vi "GetGearMainpulatorLift.vi"(11 "Gear Manipulator in":refnum<class "Gear Manipulator.lvclass">) -> (2 "Gear Mainpulator Lift":bool, 3 "Gear Manipulator out":refnum<class "Gear Manipulator.lvclass">)   [LabVIEW 2016, in "Gear Manipulator.lvclass"]
uses:
  Gear Manipulator.lvclass
  Gear Manipulator.lvclass/Gear Manipulator.ctl
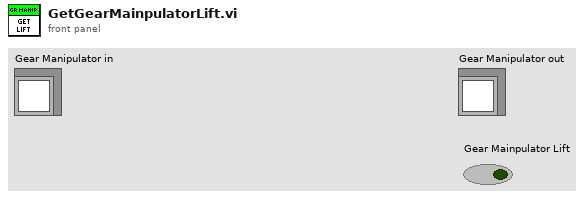
[diagram p1: front panel]
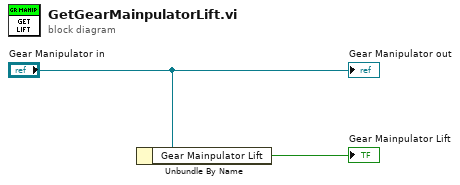
[diagram p0: block diagram]
diagram:
  n1 = Unbundle By Name("Gear Manipulator in") -> ("Gear Mainpulator Lift"=→"Gear Mainpulator Lift":bool)
  "Gear Manipulator out" <- "Gear Manipulator in"
